vi "GetQualifiedName.vi"(8 "error in (no error)":errorcluster, 11 "CLabVIEWItem in":refnum<class "CLabVIEWItem.lvclass">) -> (0 "error out":errorcluster, 1 "Qualified name":string, 3 "CLabVIEWItem out":refnum<class "CLabVIEWItem.lvclass">)   [LabVIEW 2020, in "LabVIEWItem.lvlib" / "CLabVIEWItem.lvclass"]
uses:
  CLabVIEWItem.lvclass
  CLabVIEWItem.lvclass/CLabVIEWItem.ctl
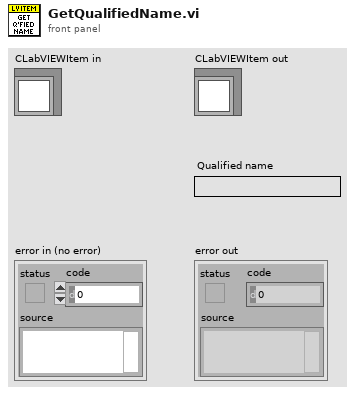
[diagram p1: front panel]
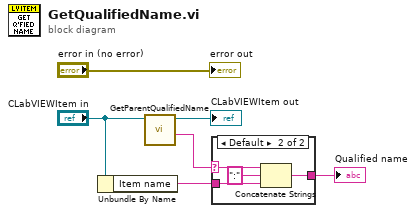
[diagram p0: block diagram]
diagram:
  n1 = Unbundle By Name("CLabVIEWItem in") -> ("Item name"=w1:string)
  n2 = call-dynamic "GetParentQualifiedName.vi"("CLabVIEWItem in"="CLabVIEWItem in") -> ("Name"=w3:string, "CLabVIEWItem out"=→"CLabVIEWItem out":refnum<class "CLabVIEWItem.lvclass">)  [unwired: 8 in, 1 out]
  n3 = case shown="Default" w3 {
    selector: w3 -> [_ w8]
    tunnel: w1 -> [w7 w11]
    tunnel: [w7 w9] -> w5
    frame "" {
    }
    frame Default {
      n4 = Concatenate Strings(w8, ":" ("delimiter (Tab)"), w11) -> (w9:string)
    }
  }
  "Qualified name" <- w5
  "error out" <- "error in (no error)"
